vi "ScaleRotVel.vi"(6 "Scale Dir":T1=enum."Full scale -> Model scale", 8 "Scale factor":dbl, 11 "Rotational Velocity (In)":dbl) -> (3 "Rotational Velocity (Out)":dbl)   [LabVIEW 2018]
uses:
  Clusters/ScalingEnum.ctl
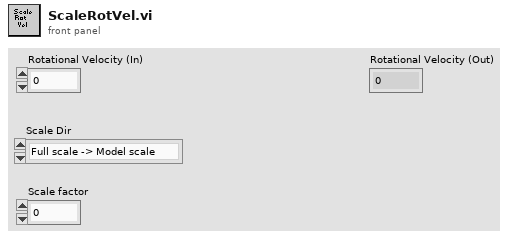
[diagram p1: front panel]
types:
  T1 = typedef "ScalingEnum.ctl" = enum16{"Model scale -> Full scale", "Full scale -> Model scale"}
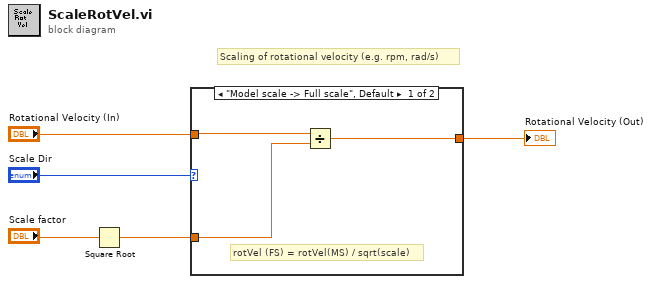
[diagram p0: block diagram]
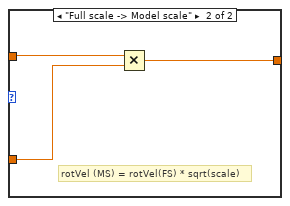
[diagram p2: hidden frame]
diagram:
  # "Scaling of rotational velocity (e.g. rpm, rad/s)"
  n1 = Square Root(x="Scale factor") -> (sqrt(x)=w2:dbl)
  n2 = case shown="\"Model scale -> Full scale\", Default" "Scale Dir" {
    tunnel: "Rotational Velocity (In)" -> [w8 w11]
    tunnel: w2 -> [w7 w10]
    tunnel: [w6 w9] -> w1
    frame "Model scale -> Full scale", Default {
      # "rotVel (FS) = rotVel(MS) / sqrt(scale)"
      n3 = Divide(x=w8, y=w7) -> (x/y=w6:dbl)
    }
    frame "Full scale -> Model scale" {
      # "rotVel (MS) = rotVel(FS) * sqrt(scale)"
      n4 = Multiply(x=w11, y=w10) -> (x*y=w9:dbl)
    }
  }
  "Rotational Velocity (Out)" <- w1
